vi "EChem Signal.vi"(0 "V_Zeta in":dbl, 1 "Capacitance Functional Molecules per NS":dbl, 2 "Series Resistance of Solution":dbl, 3 "Frequency":dbl, 4 "Freq Hz-MHz":dbl, 5 "Capacitance Functional Analyte per NS":dbl, 8 "C_EDL/ 1 NS":dbl) -> (12 "Impedance of EDL & Functionalization & Analyte":dbl, 14 "Impedance of EDL & Functionalization":dbl, 15 "Capacitance of ELD & Functionalization":dbl, 16 "Total Impedance Rs+C(EDS+Funct)":dbl, 17 "Capacitance of ELD & Functionalization & Analyte":dbl, 18 "Total Impedance Rs+C(EDS+Funct+Analyte)":dbl, 19 "Delta C":dbl, 20 "Delta Total Impedance":dbl, 21 "V_Zeta out":dbl, 22 "Max i;  R+ C (EDL+Funct)":dbl format="%#_9e", 23 "|Z| of R+ C (EDL+Funct)":dbl, 24 "Delta i":dbl, 25 "Max i;  R+ C (EDL+Funct+ Analyte)":dbl format="%#_9e", 26 "|Z| of R+ C (EDL+Funct+Analyte)":dbl)   [LabVIEW 2020]
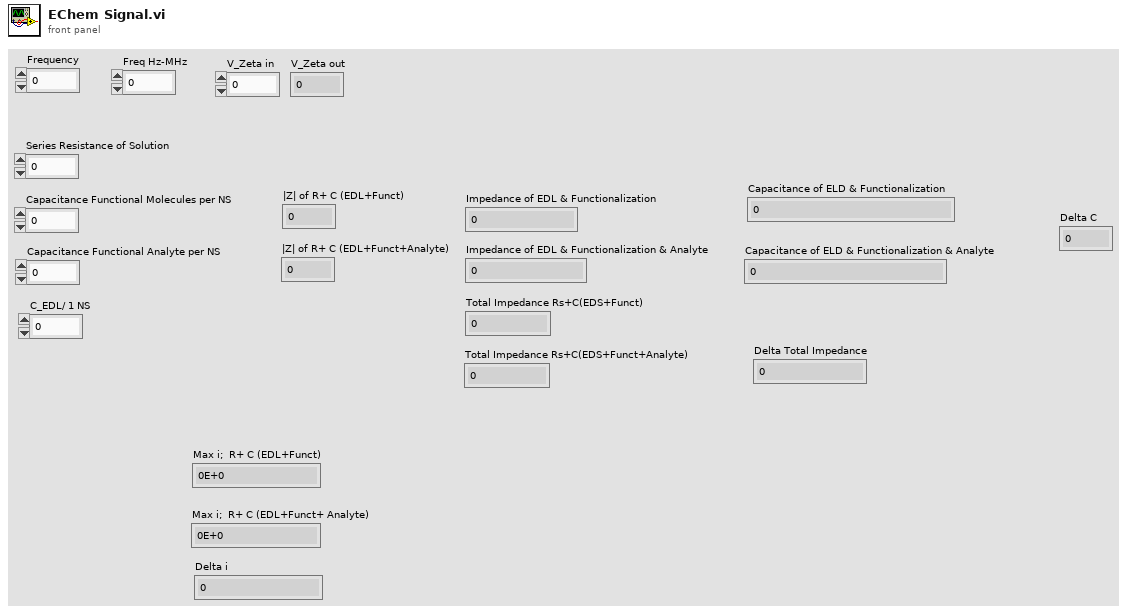
[diagram p1: front panel]
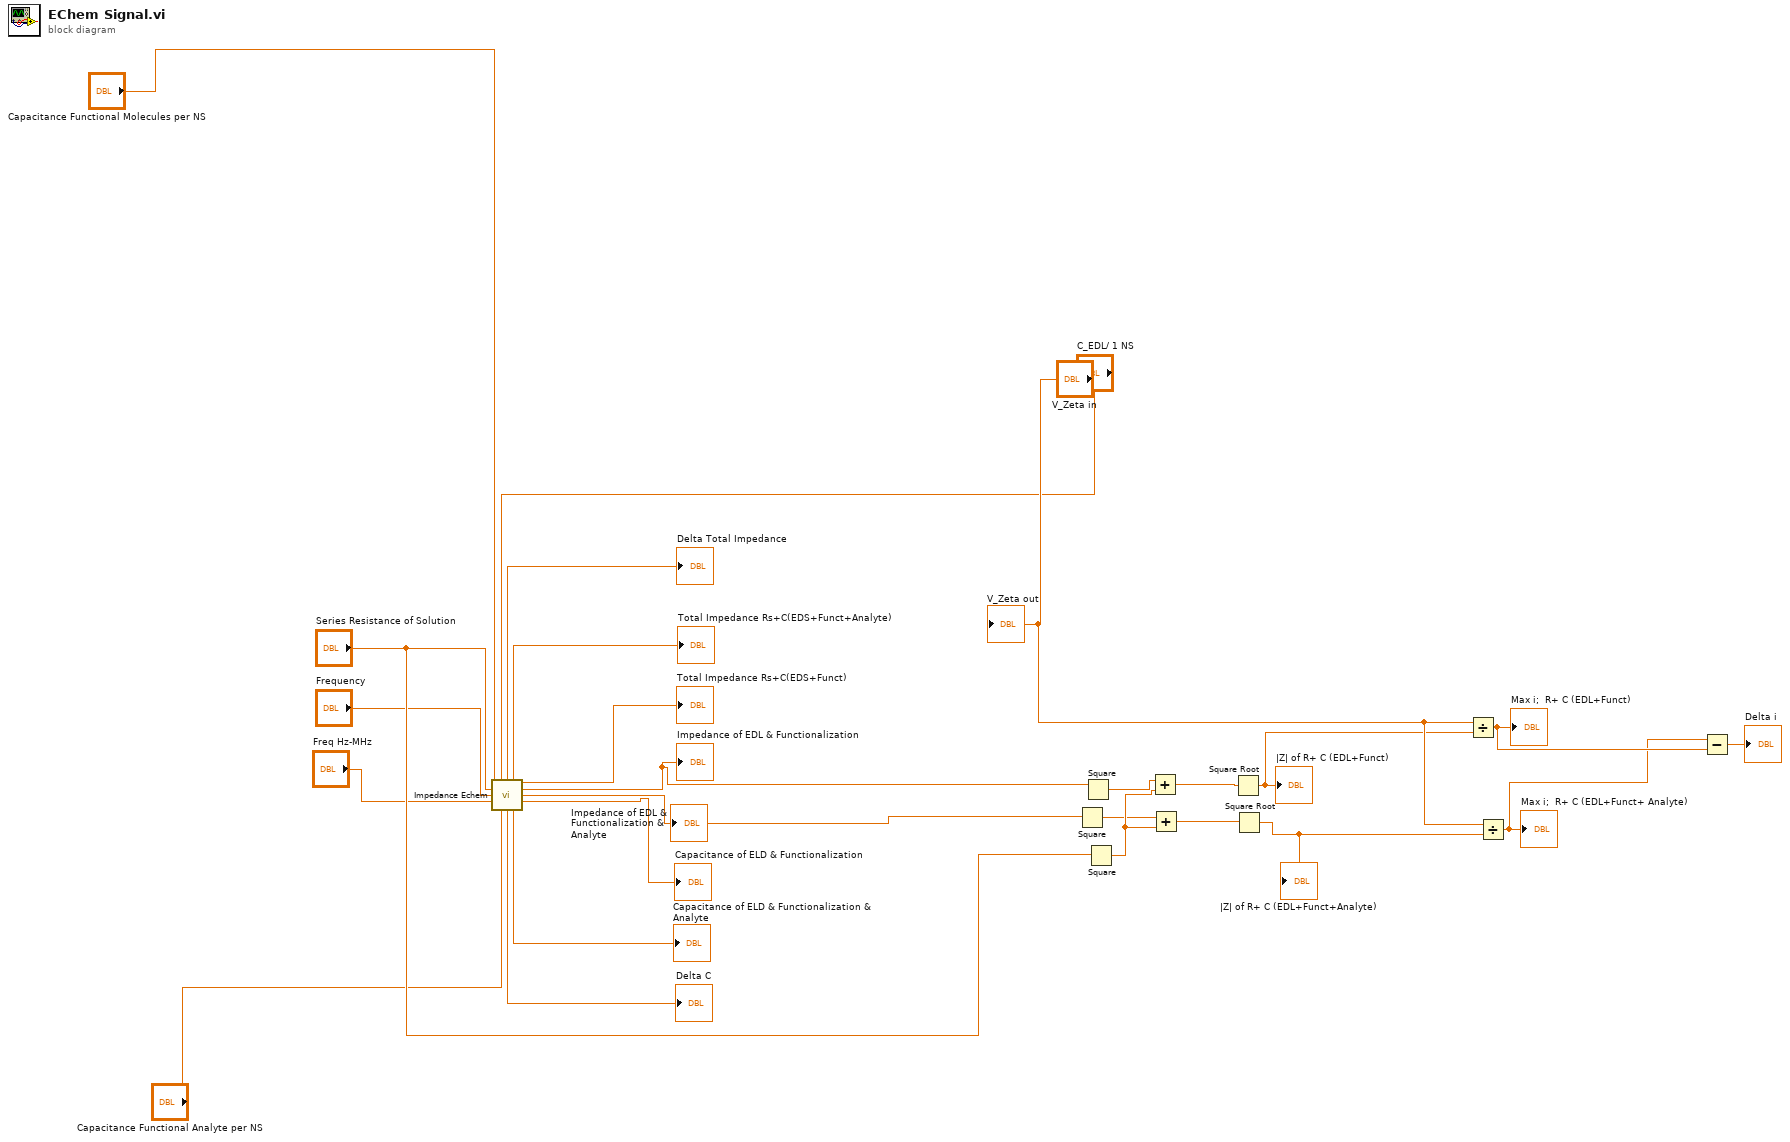
[diagram p0: block diagram]
diagram:
  n1 = call "Impedance Echem.vi"("Capacitance Functional Molecules per NS"="Capacitance Functional Molecules per NS", "C_EDL/ 1 NS"="C_EDL/ 1 NS", "Series Resistance of Solution"="Series Resistance of Solution", "Frequency"="Frequency", "Freq Hz-MHz"="Freq Hz-MHz", "Capacitance Functional Analyte per NS"="Capacitance Functional Analyte per NS") -> ("Delta Total Impedance"=→"Delta Total Impedance":dbl, "Total Impedance Rs+C(EDS+Funct+Analyte)"=→"Total Impedance Rs+C(EDS+Funct+Analyte)":dbl, "Total Impedance Rs+C(EDS+Funct)"=→"Total Impedance Rs+C(EDS+Funct)":dbl, "Impedance of EDL & Functionalization"=w13:dbl, "Impedance of EDL & Functionalization & Analyte"=w14:dbl, "Capacitance of ELD & Functionalization"=→"Capacitance of ELD & Functionalization":dbl, "Delta C"=→"Delta C":dbl, "Capacitance of ELD & Functionalization & Analyte"=→"Capacitance of ELD & Functionalization & Analyte":dbl)  [unwired: 2 in]
  "Impedance of EDL & Functionalization" <- w13
  "Impedance of EDL & Functionalization & Analyte" <- w14
  n2 = Square(x=w14) -> (x^2=w16:dbl)
  n3 = Square(x=w13) -> (x^2=w15:dbl)
  n4 = Square(x="Series Resistance of Solution") -> (x^2=w17:dbl)
  n5 = Add(x=w15, y=w17) -> (x+y=w18:dbl)
  n6 = Add(x=w16, y=w17) -> (x+y=w19:dbl)
  n7 = Square Root(x=w18) -> (sqrt(x)=w20:dbl)
  "|Z| of R+ C (EDL+Funct)" <- w20
  n8 = Square Root(x=w19) -> (sqrt(x)=w21:dbl)
  "|Z| of R+ C (EDL+Funct+Analyte)" <- w21
  n9 = Divide(x="V_Zeta in", y=w20) -> (x/y=w24:dbl)
  "Max i;  R+ C (EDL+Funct)" <- w24
  n10 = Divide(x="V_Zeta in", y=w21) -> (x/y=w23:dbl)
  "Max i;  R+ C (EDL+Funct+ Analyte)" <- w23
  n11 = Subtract(x=w23, y=w24) -> (x-y=→"Delta i":dbl)
  "V_Zeta out" <- "V_Zeta in"
